vi "ConfigParams - Parse - General.vi"(8 "error in (no error)":errorcluster, 11 "Ethernet in":refnum<class "ENET_BS1201.lvclass">) -> (0 "error out":errorcluster, 1 "Firmware":string, 2 "IPAddress":string, 3 "Ethernet out":refnum<class "ENET_BS1201.lvclass">)   [LabVIEW 2021, in "BS120x Driver.lvlib" / "ENET_BS1201.lvclass"]
uses:
  ENET_BS1201.lvclass
panel:
  # "[General]\nIPAddress = %s\nFirmware = %s"
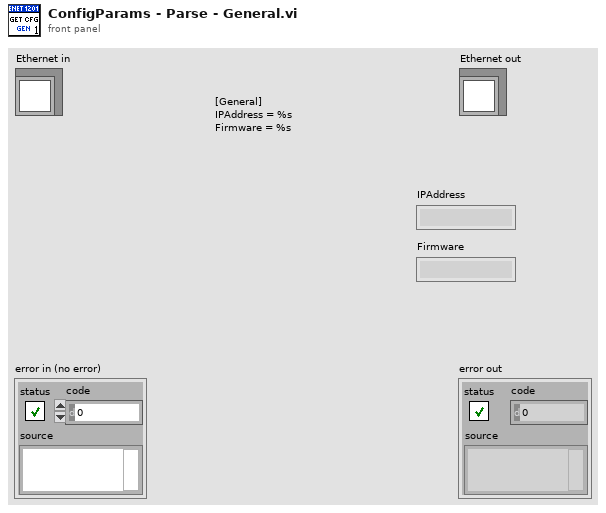
[diagram p1: front panel]
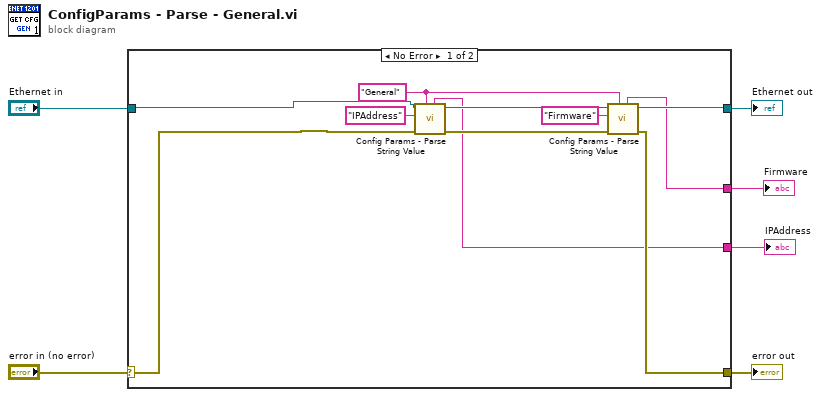
[diagram p0: block diagram]
diagram:
  n1 = case shown="No Error" "error in (no error)" {
    selector: "error in (no error)" -> [w10 w19]
    tunnel: [w11 w19] -> w5
    tunnel: [w12 w18] -> w3
    tunnel: "Ethernet in" -> [w9 w18]
    tunnel: [w8 _] -> w2
    tunnel: [w7 _] -> w1
    frame No Error {
      w14 = "General" ("Section")
      n2 = call-dynamic "Config Params - Parse String Value.vi"("Section"=w14, "error in (no error)"=w10, "Key"="IPAddress", "Ethernet in"=w9) -> ("error out"=w15:errorcluster, "Ethernet out"=w16:refnum<class "ENET_BS1201.lvclass">, "Value (str)"=w8:string)  [unwired: 1 in, 4 out]
      n3 = call-dynamic "Config Params - Parse String Value.vi"("Section"=w14, "error in (no error)"=w15, "Key"="Firmware", "Ethernet in"=w16) -> ("error out"=w11:errorcluster, "Ethernet out"=w12:refnum<class "ENET_BS1201.lvclass">, "Value (str)"=w7:string)  [unwired: 1 in, 4 out]
    }
    frame Error {
    }
  }
  "error out" <- w5
  "Ethernet out" <- w3
  "IPAddress" <- w2
  "Firmware" <- w1
